vi "Build String.vi"(7 "Section":string[](array[string]), 8 "error in (no error)":errorcluster, 9 "Values":string[](array[string]), 10 "Keys":string[](array[string]), 11 "ConfigManager.Text in":refnum<class "ConfigManager.Text.lvclass">) -> (0 "error out":errorcluster, 2 "Input String":string, 3 "ConfigManager.Text out":refnum<class "ConfigManager.Text.lvclass">)   [LabVIEW 2013, in "CfgManager.Text.lvlib" / "ConfigManager.Text.lvclass"]
uses:
  ConfigManager.Text.lvclass
  ConfigManager.Text.lvclass/ConfigManager.Text.ctl
  <vilib>/LabVIEW Open Source Project/Unicity/Delimiter/Delimiter.lvclass
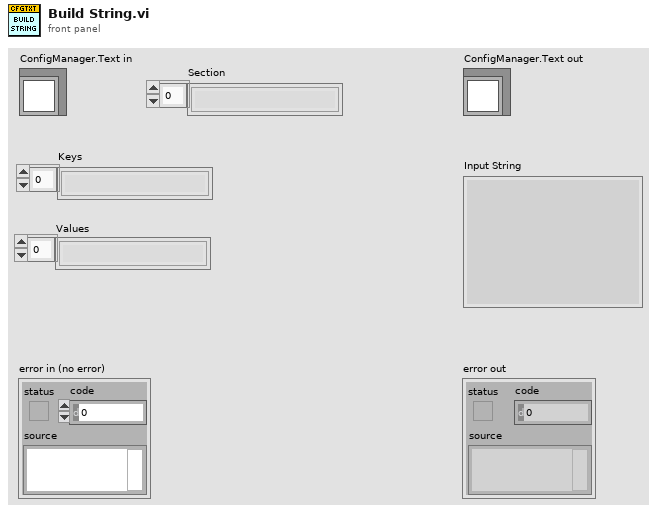
[diagram p1: front panel]
types:
  T1 = typedef "CfgManager.Text.lvlib/ConfigManager.Text.lvclass/Configuration -- Cluster.ctl" = cluster{"FileHeader":refnum<class "FileHeader.lvclass">, "FileSignature":refnum<class "FileSignature.lvclass">, "Section Delimiter":refnum<class "Delimiter.lvclass">, "Key-Value Separator":refnum<class "Delimiter.lvclass">}
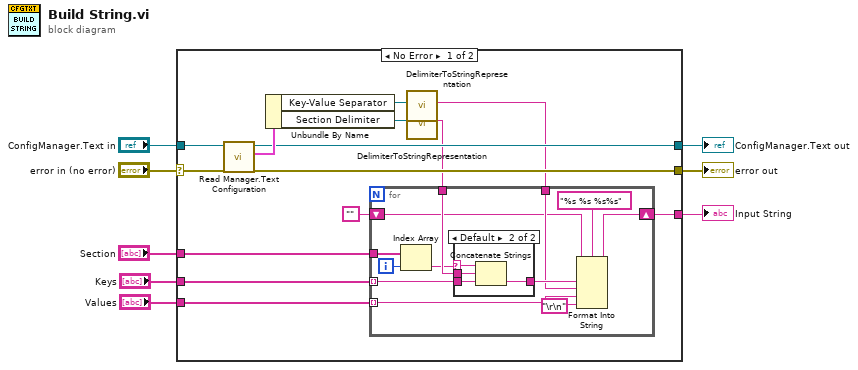
[diagram p0: block diagram]
diagram:
  n1 = case shown="No Error" "error in (no error)" {
    selector: "error in (no error)" -> [w21 w40]
    tunnel: [w21 w40] -> w7
    tunnel: [w17 w39] -> w5
    tunnel: "ConfigManager.Text in" -> [w20 w39]
    tunnel: "Section" -> [w14 _]
    tunnel: "Keys" -> [w13 _]
    tunnel: "Values" -> [w12 _]
    tunnel: [w9 _] -> w1
    frame No Error {
      n2 = call "Read Manager.Text Configuration.vi"("ConfigManager.Text in"=w20) -> ("Manager.Text Configuration"=w19:T1, "ConfigManager.Text out"=w17:refnum<class "ConfigManager.Text.lvclass">)  [unwired: 9 in]
      n3 = Unbundle By Name(w19) -> ("Key-Value Separator"=w16:refnum<class "Delimiter.lvclass">, "Section Delimiter"=w18:refnum<class "Delimiter.lvclass">)
      n4 = call <vilib>:"DelimiterToStringRepresentation.vi"("Delimiter"=w16) -> ("String representation"=w10:string)  [unwired: 10 in]
      n5 = call <vilib>:"DelimiterToStringRepresentation.vi"("Delimiter"=w18) -> ("String representation"=w11:string)  [unwired: 10 in]
      n6 = for {
        shift-right: [w26] -> w9
        shift-left: "" -> [w27]
        tunnel: w14 -> [w23]
        tunnel: w13 -> [w32] mode=indexing
        tunnel: w12 -> [w29] mode=indexing
        tunnel: w11 -> [w33]
        tunnel: w10 -> [w30]
        i -> [w24]
        n7 = Index Array(array=w23, index=w24) -> (element=w22:string)
        n8 = case shown="Default" w22 {
          selector: w22 -> [_ w38]
          tunnel: w33 -> [_ w37]
          tunnel: w32 -> [w34 w36]
          tunnel: [w34 w35] -> w31
          frame "\u0000" {
          }
          frame Default {
            n9 = Concatenate Strings(w38, w37, w36) -> (w35:string)
          }
        }
        n10 = Format Into String(format string="%s %s %s%s", initial string=w27, w31, w30, w29, "\r\n") -> (resulting string=w26:string)  [unwired: 1 in, 1 out]
      }
    }
    frame Error {
    }
  }
  "error out" <- w7
  "ConfigManager.Text out" <- w5
  "Input String" <- w1
